vi "MAINP Get DBECUs.vi"(8 "error in (no error)":errorcluster, 10 "Alias":string, 11 "Device Item Ref in":T1 format="%.0x") -> (0 "error out":errorcluster, 1 "ECU":string, 2 "Cluster":string, 3 "Device Item Ref out":T1 format="%.0x")   [LabVIEW 2018, in "CAN Gateway System Explorer.lvlib"]
uses:
  CAN Gateway System Explorer.lvlib
  <vilib>/NI Veristand/Custom Device API/Custom Device Item Ref.ctl
  <resource>/objmgr/xnet.rc
  <vilib>/NI Veristand/Custom Device API/Custom Device API.lvlib
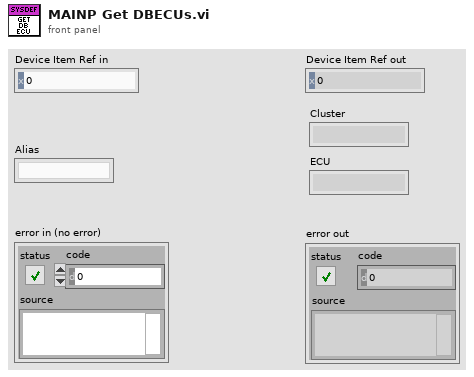
[diagram p1: front panel]
types:
  T1 = typedef "Custom Device API.lvlib/Custom Device Item Ref.ctl" = u64
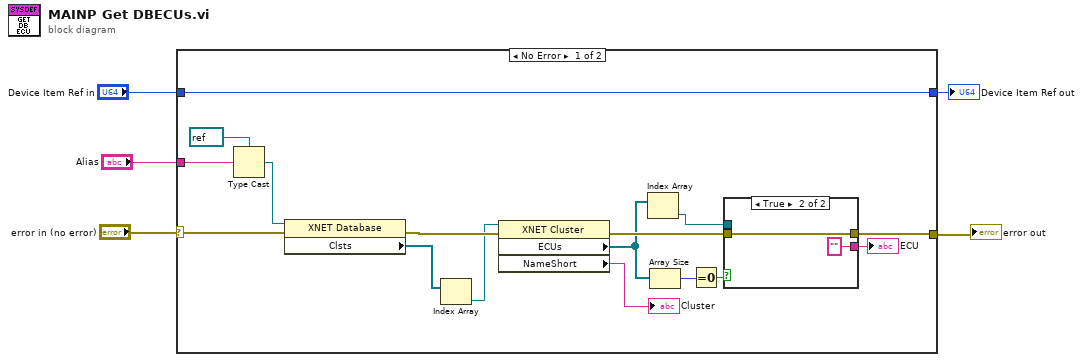
[diagram p0: block diagram]
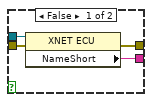
[diagram p2: hidden frame]
diagram:
  n1 = case shown="No Error" "error in (no error)" {
    selector: "error in (no error)" -> [w19 w29]
    tunnel: "Device Item Ref in" -> [w21 w28]
    tunnel: [w21 w28] -> w3
    tunnel: [w15 w29] -> w2
    tunnel: "Alias" -> [w20 _]
    frame No Error {
      n2 = Type Cast(type=refnum<k21> refnum ("XNET Database"), x=w20) -> (*(type *) &x=w17:refnum<k21>)
      n3 = property class="XNET Database"(reference=w17, error in=w19) -> (error out=w16:errorcluster, "Clsts"=w13:refnum<k21>[])  [unwired: 1 out]
      n4 = Index Array(array=w13) -> (element=w12:refnum<k21>)  [unwired: 1 in]
      n5 = property class="XNET Cluster"(reference=w12, error in=w16) -> (error out=w14:errorcluster, "ECUs"=w7:refnum<k21>[], "NameShort"=→"Cluster":string)  [unwired: 1 out]
      n6 = Index Array(array=w7) -> (element=w6:refnum<k21>)  [unwired: 1 in]
      n7 = Array Size(array=w7) -> (size(s)=w10:i32)
      n8 = Equal To 0?(x=w10) -> (x = 0?=w9:bool)
      n9 = case shown="True" w9 {
        tunnel: [w25 w27] -> w15
        tunnel: w14 -> [w24 w27]
        tunnel: [w23 "" ("NameShort")] -> w8
        tunnel: w6 -> [w22 _]
        frame False {
          n10 = property class="XNET ECU"(reference=w22, error in=w24) -> (error out=w25:errorcluster, "NameShort"=w23:string)  [unwired: 1 out]
        }
        frame True {
        }
      }
      "ECU" <- w8
    }
    frame Error {
    }
  }
  "error out" <- w2
  "Device Item Ref out" <- w3
